vi "FindChannelParams.vi"(7 "index":i32, 8 "error in":errorcluster, 9 "ChannelParams":T1[](array[typedef]), 10 "Direction":T5(ring), 11 "ChannelNumber":u8) -> (0 "error out":errorcluster, 2 "LabelParams":T2[](array[typedef]), 3 "Found":bool)   [LabVIEW 2016]
uses:
  Controls/LabelParam.ctl
  Controls/LabelInfo.ctl
  Controls/ARINCParam.ctl
  Controls/ChannelParams.ctl
  Ballard Arinc-429 System Explorer.lvlib
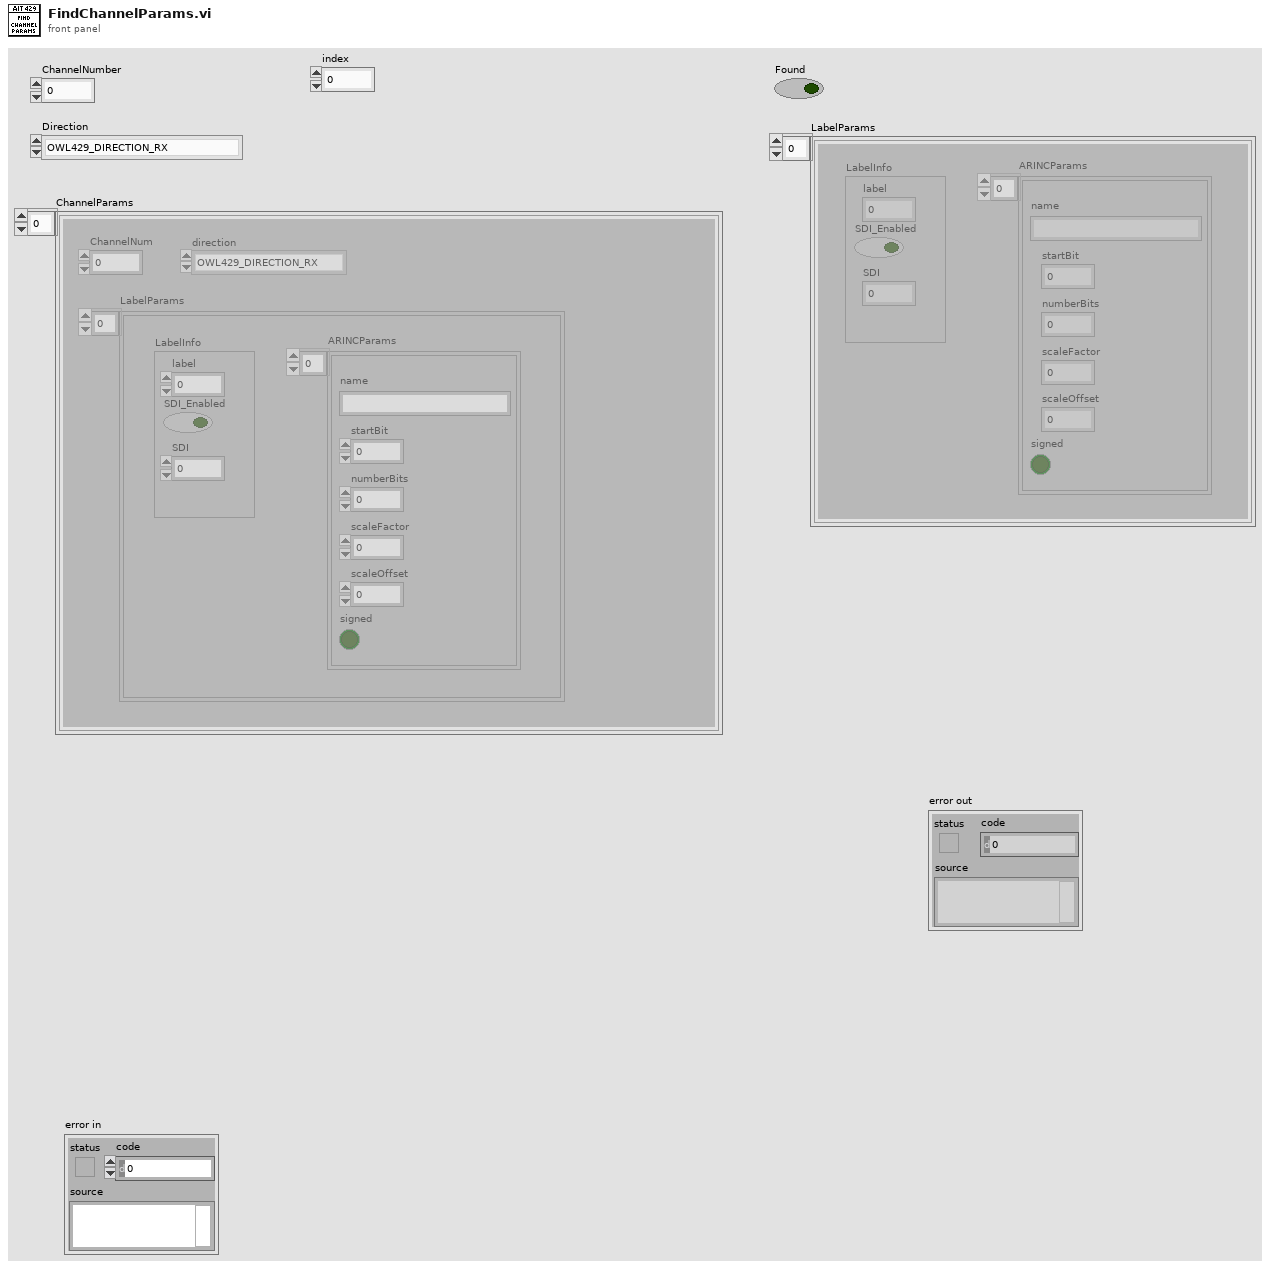
[diagram p1: front panel]
types:
  T1 = typedef "Ballard Arinc-429 System Explorer.lvlib/ChannelParams.ctl" = cluster{"ChannelNum":u8, "LabelParams":T2[], "direction":enum16{"OWL429_DIRECTION_RX", "OWL429_DIRECTION_TX"}}
  T2 = typedef "Ballard Arinc-429 System Explorer.lvlib/LabelParam.ctl" = cluster{"LabelInfo":T3, "ARINCParams":T4[]}
  T3 = typedef "Ballard Arinc-429 System Explorer.lvlib/LabelInfo.ctl" = cluster{"label":u32, "SDI_Enabled":bool, "SDI":u8}
  T4 = typedef "Ballard Arinc-429 System Explorer.lvlib/ARINCParam.ctl" = cluster{"name":string, "startBit":i32, "numberBits":i32, "scaleFactor":dbl, "scaleOffset":dbl, "signed":bool}
  T5 = enum16{"OWL429_DIRECTION_RX", "OWL429_DIRECTION_TX"}
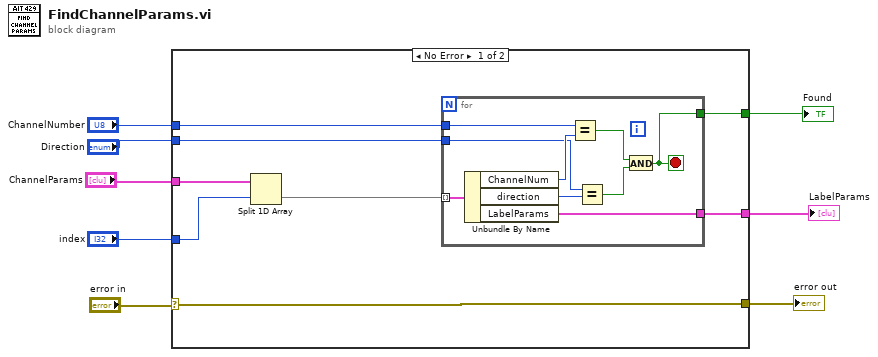
[diagram p0: block diagram]
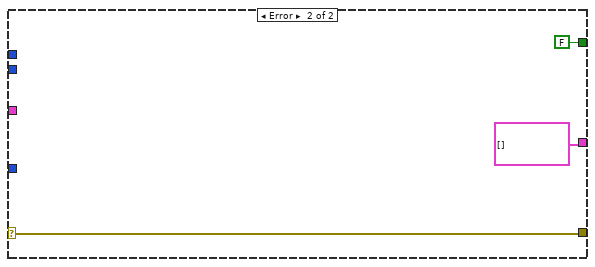
[diagram p2: hidden frame]
diagram:
  n1 = case shown="No Error" "error in" {
    selector: "error in" -> [w9 w28]
    tunnel: "index" -> [w16 _]
    tunnel: "ChannelParams" -> [w15 _]
    tunnel: [w13 FALSE] -> w7
    tunnel: [w12 T2[] [] ("LabelParams")] -> w6
    tunnel: "Direction" -> [w11 _]
    tunnel: "ChannelNumber" -> [w10 _]
    tunnel: [w9 w28] -> w2
    frame No Error {
      n2 = Split 1D Array(array=w15, index=w16) -> (second subarray=w14:T1[])  [unwired: 1 out]
      n3 = for {
        tunnel: w14 -> [w23] mode=indexing
        tunnel: w10 -> [w25]
        tunnel: w11 -> [w22]
        tunnel: [w19] -> w13
        tunnel: [w17] -> w12
        stop <- w19 stop-if-true
        n4 = Unbundle By Name(w23) -> ("ChannelNum"=w24:u8, "direction"=w18:T5, "LabelParams"=w17:T2[])
        n5 = Equal?(x=w25, y=w24) -> (x = y?=w21:bool)
        n6 = Equal?(x=w22, y=w18) -> (x = y?=w20:bool)
        n7 = And(x=w21, y=w20) -> (x .and. y?=w19:bool)
      }
    }
    frame Error {
    }
  }
  "Found" <- w7
  "LabelParams" <- w6
  "error out" <- w2
